vi "Read_ini_AllArrayStr.vi"(0 "configuration file path":path) -> (1 "Section":string[](array[string]), 2 "Value":string[][](array[string]))   [LabVIEW 2015]
uses:
  <vilib>/Utility/config.llb/Read Key (String).vi
  <vilib>/Utility/config.llb/NI_LVConfig.lvlib
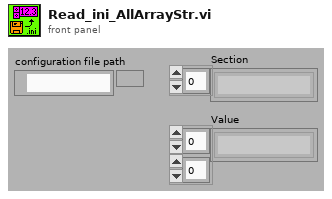
[diagram p1: front panel]
types:
  T1 = typedef "NI_LVConfig.lvlib/Config Data RefNum.ctl" = refnum<k1>
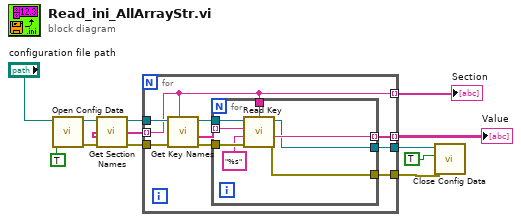
[diagram p0: block diagram]
diagram:
  n1 = call <vilib>:"Open Config Data.vi"("create file if necessary (T)"=TRUE ("create file if necessary? (T)"), "configuration file path"="configuration file path") -> ("error out"=w3:errorcluster, "refnum"=w4:T1)  [unwired: 7 in, 1 out]
  n2 = call <vilib>:"Get Section Names.vi"("error in (no error)"=w3, "refnum"=w4) -> ("error out"=w5:errorcluster, "section names"=w7:string[], "refnum out"=w6:T1)  [unwired: 7 in]
  n3 = for {
    tunnel: w5 -> [w21]
    tunnel: w6 -> [w20]
    tunnel: w7 -> [w13] mode=indexing
    tunnel: [w17] -> w11 mode=indexing
    tunnel: [w15] -> w8
    tunnel: [w14] -> w9
    tunnel: [w13] -> w1 mode=indexing
    n4 = call <vilib>:"Get Key Names.vi"("section"=w13, "error in (no error)"=w21, "refnum"=w20) -> ("error out"=w19:errorcluster, "key names"=w18:string[], "refnum out"=w16:T1)  [unwired: 5 in, 1 out]
    n5 = for {
      tunnel: w19 -> [w29]
      tunnel: w18 -> [w28] mode=indexing
      tunnel: w13 -> [w27]
      tunnel: [w26] -> w17 mode=indexing
      tunnel: w16 -> [w25]
      tunnel: [w24] -> w15
      tunnel: [w23] -> w14
      n6 = call-poly <vilib>:"Read Key.vi"("section"=w27, "error in (no error)"=w29, "default value"="%s", "key"=w28, "refnum"=w25) -> ("error out"=w23:errorcluster, "value"=w26:string, "refnum out"=w24:T1)  [unwired: 3 in, 1 out]
    }
  }
  "Value" <- w11
  "Section" <- w1
  n7 = call <vilib>:"Close Config Data.vi"("error in (no error)"=w9, "write file if changed (T)"=TRUE ("write configuration file? (T)"), "refnum"=w8) -> ()  [unwired: 7 in, 2 out]
